vi "Launch Nested Actors.vi"(8 "error in":errorcluster, 11 "Platform in":refnum<class "Platform.lvclass">) -> (0 "error out":errorcluster, 3 "Platform out":refnum<class "Platform.lvclass">)   [LabVIEW 2019, in "Platform.lvlib" / "Platform.lvclass"]
uses:
  Platform.lvclass
  C:/Program Files (x86)/National Instruments/LabVIEW 2019/vi.lib/ActorFramework/Actor/Actor.lvclass
  Sequence/Sequence/Sequence.lvclass
  Timer/Timer/Timer.lvclass
  Platform Messages/Receive Seq Msg/Receive Seq Msg.lvclass
  C:/Working Copy/trunk/Modified Cobra Jung/Cobra/Cobra AF/Sequence/Sequence Messages/Sequence Msg/Sequence Msg.lvclass
  Platform Messages/Receive Time Info Msg/Receive Time Info Msg.lvclass
  C:/Working Copy/trunk/Modified Cobra Jung/Cobra/Cobra AF/Timer/Timer Messages/Time Info Msg/Time Info Msg.lvclass
  Timer/Timer/Timer.lvclass/Timer.ctl
  Sequence/Sequence/Sequence.lvclass/Sequence.ctl
  Platform.lvclass/Platform.ctl
  <vilib>/ActorFramework/Actor/Actor.lvclass
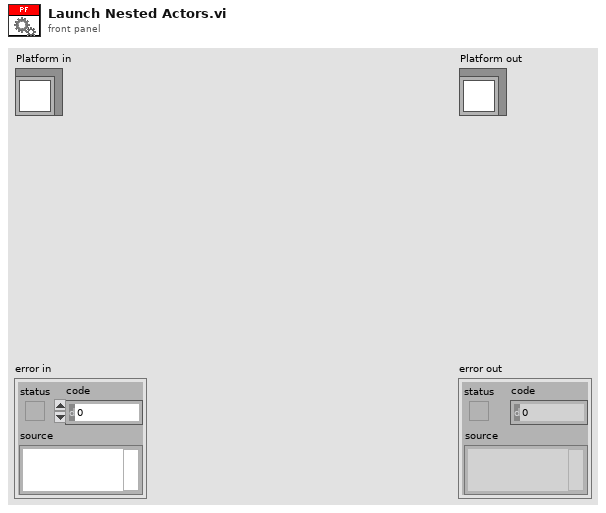
[diagram p1: front panel]
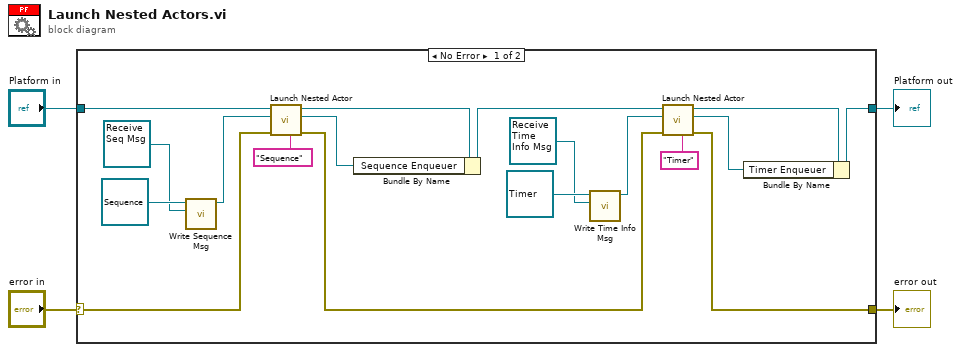
[diagram p0: block diagram]
diagram:
  n1 = case shown="No Error" "error in" {
    selector: "error in" -> [w21 w24]
    tunnel: [w5 w24] -> w3
    tunnel: [w6 w23] -> w1
    tunnel: "Platform in" -> [w22 w23]
    frame No Error {
      n2 = call "Write Sequence Msg.vi"("Sequence.lvlib:Sequence Msg.lvclass"=refnum<class "Receive Seq Msg.lvclass"> refnum ("TTV Test.lvlib:Receive Seq Msg.lvclass"), "Sequence in"=refnum<class "Sequence.lvclass"> refnum ("Sequence.lvlib:Sequence.lvclass")) -> ("Sequence out"=w11:refnum<class "Sequence.lvclass">)  [unwired: 9 in]
      n3 = call <vilib>:"Launch Nested Actor.vi"("Debug Alias"="Sequence", "error in (no error)"=w21, "Nested Actor"=w11, "Caller Actor in"=w22) -> ("error out"=w18:errorcluster, "Nested Actor's Enqueuer"=w16:refnum<class "Message Enqueuer.lvclass">, "Caller Actor out"=w17:refnum<class "Platform.lvclass">)  [unwired: 5 in]
      n4 = Bundle By Name(cluster=w17, "Sequence Enqueuer"=w16) -> (w15:refnum<class "Platform.lvclass">)
      n5 = call "Write Time Info Msg.vi"("Timer.lvlib:Time Info Msg.lvclass"=refnum<class "Receive Time Info Msg.lvclass"> refnum ("TTV Test.lvlib:Receive Time Info Msg.lvclass"), "Timer in"=refnum<class "Timer.lvclass"> refnum ("Timer.lvlib:Timer.lvclass")) -> ("Timer out"=w7:refnum<class "Timer.lvclass">)  [unwired: 9 in]
      n6 = call <vilib>:"Launch Nested Actor.vi"("Debug Alias"="Timer", "error in (no error)"=w18, "Nested Actor"=w7, "Caller Actor in"=w15) -> ("error out"=w5:errorcluster, "Nested Actor's Enqueuer"=w13:refnum<class "Message Enqueuer.lvclass">, "Caller Actor out"=w14:refnum<class "Platform.lvclass">)  [unwired: 5 in]
      n7 = Bundle By Name(cluster=w14, "Timer Enqueuer"=w13) -> (w6:refnum<class "Platform.lvclass">)
    }
    frame Error {
    }
  }
  "error out" <- w3
  "Platform out" <- w1
